vi "Run Headless.vi"(8 "error in (no error)":errorcluster, 10 "Mediator Type":refnum<class "IMediator.lvclass">, 11 "RootModel in":refnum<class "RootModel.lvclass">) -> (0 "error out":errorcluster, 3 "RootModel out":refnum<class "RootModel.lvclass">)   [LabVIEW 2017, in "RootModel.lvlib" / "RootModel.lvclass"]
uses:
  <vilib>/gpm_packages/@cs/mva-core/Source/RootModel/RootModel/RootModel.lvclass
  C:/Program Files/National Instruments/LabVIEW 2017/vi.lib/ActorFramework/Actor/Actor.lvclass
  C:/Program Files/National Instruments/LabVIEW 2017/vi.lib/gpm_packages/@cs/mva-core/Source/IObserver/IObserver/IObserver.lvclass
  C:/Program Files/National Instruments/LabVIEW 2017/vi.lib/gpm_packages/@cs/mva-core/Source/IModel/IModel/IModel.lvclass
  <vilib>/gpm_packages/@cs/mva-core/Source/IMediator/IMediator/IMediator.lvclass
  <vilib>/gpm_packages/@cs/mva-core/Source/IObserver/IObserver/IObserver.lvclass/IObserver.ctl
  <vilib>/gpm_packages/@cs/mva-core/Source/IModel/IModel/IModel.lvclass/IModel.ctl
  <vilib>/gpm_packages/@cs/mva-core/Source/IModel/IModel/IModel.lvclass
  <vilib>/ActorFramework/Actor/Actor.lvclass
  <vilib>/gpm_packages/@cs/mva-core/Source/IObserver/IObserver/IObserver.lvclass
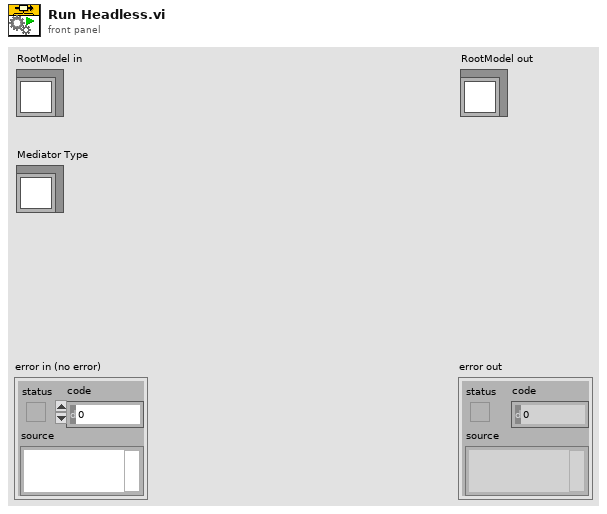
[diagram p1: front panel]
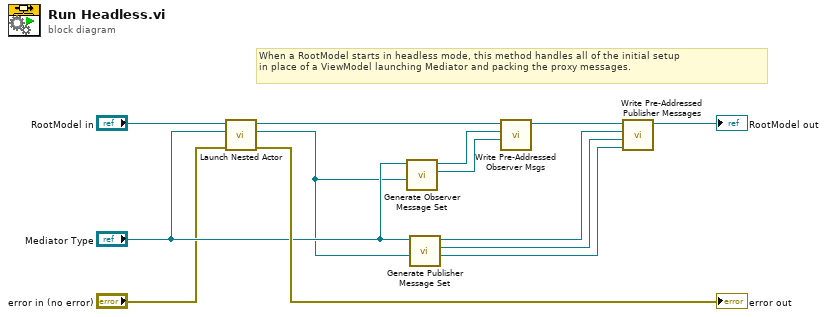
[diagram p0: block diagram]
diagram:
  # "When a RootModel starts in headless mode, this method handles all of the initial setup\nin place of a ViewModel launching Mediator and packing the proxy messages."
  n1 = call <vilib>:"Launch Nested Actor.vi"("error in (no error)"="error in (no error)", "Nested Actor"="Mediator Type", "Caller Actor in"="RootModel in") -> ("error out"=→"error out":errorcluster, "Nested Actor's Enqueuer"=w1:refnum<class "Message Enqueuer.lvclass">, "Caller Actor out"=w12:refnum<class "RootModel.lvclass">)  [unwired: 6 in]
  n2 = call-dynamic "Generate Observer Message Set.vi"("Mediator Enqueuer"=w1, "Mediator Type"="Mediator Type") -> ("Unsubscribe Msg"=w8:refnum<class "Unsubscribe Msg.lvclass">, "Subscribe Msg"=w9:refnum<class "Subscribe Msg.lvclass">)  [unwired: 8 in]
  n3 = call-dynamic "Generate Publisher Message Set.vi"("Mediator Enqueuer"=w1, "IMediator in"="Mediator Type") -> ("Unlock Publication Msg"=w5:refnum<class "Unlock Publication Msg.lvclass">, "Lock Publication Msg"=w4:refnum<class "Lock Publication Msg.lvclass">, "Publish Msg"=w6:refnum<class "Publish Msg.lvclass">)  [unwired: 7 in]
  n4 = call <vilib>:"Write Pre-Addressed Observer Msgs.vi"("Pre-Addressed Unsubscribe Msg"=w8, "Pre-Addressed Subscribe Msg"=w9, "IObserver In"=w12) -> ("IObserver Out"=w11:refnum<class "RootModel.lvclass">)  [unwired: 8 in]
  n5 = call <vilib>:"Write Pre-Addressed Publisher Messages.vi"("Pre-Addressed Unlock Publication Msg"=w5, "Pre-Addressed Lock Publication Msg"=w4, "Pre-Addressed Publish Msg"=w6, "IModel in"=w11) -> ("IModel out"=→"RootModel out":refnum<class "RootModel.lvclass">)  [unwired: 7 in]
